vi "Array Non Decreasing.vi"(1 "array":dbl[](array[numeric])) -> (0 "Non Decreasing?":bool)   [LabVIEW 2019]
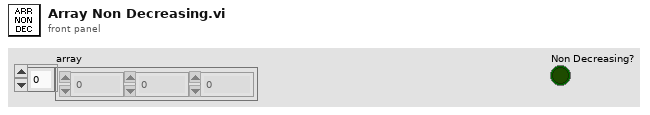
[diagram p1: front panel]
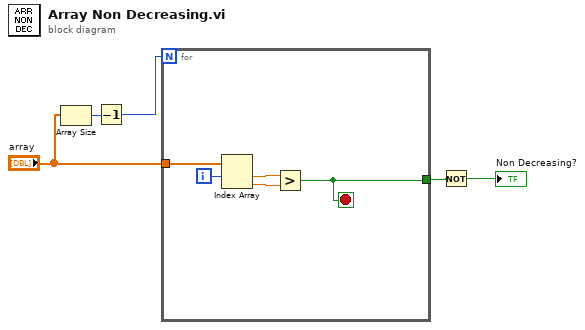
[diagram p0: block diagram]
diagram:
  n1 = Array Size(array="array") -> (size(s)=w5:i32)
  n2 = Decrement(x=w5) -> (x-1=w4:i32)
  n3 = for {
    N: w4 -> [_]
    tunnel: "array" -> [w10]
    tunnel: [w6] -> w2
    i -> [w9]
    stop <- w6 stop-if-true
    n4 = Index Array(array=w10, index #1=w9) -> (element #1=w8:dbl, element #2=w7:dbl)  [unwired: 1 in]
    n5 = Greater?(x=w8, y=w7) -> (0:w6:bool)
  }
  n6 = Not(x=w2) -> (.not. x?=→"Non Decreasing?":bool)
